vi "RegisterTrack.vi"(6 "Track ID":u64, 7 "Track Name":string, 8 "error in":errorcluster) -> (0 "error out":errorcluster)   [LabVIEW 2024, in "VS_Perfetto.lvlib"]
uses:
  VS_Perfetto.lvlib
  libvs_perfetto.dll
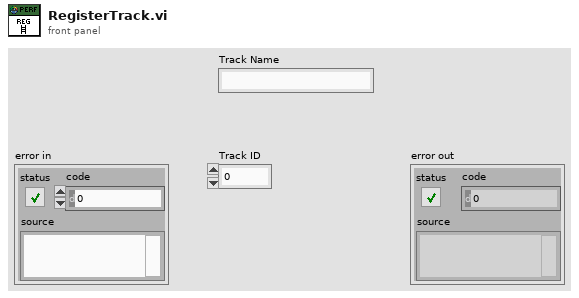
[diagram p1: front panel]
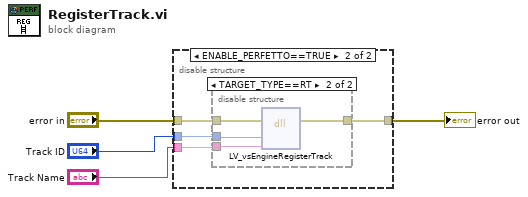
[diagram p0: block diagram]
diagram:
  n1 = disable-structure shown="ENABLE_PERFETTO==TRUE" {
    disable-tunnel: "Track Name" -> [_ w7]
    disable-tunnel: "error in" -> [w5 w8]
    disable-tunnel: [w5 w9] -> w3
    disable-tunnel: "Track ID" -> [_ w6]
    frame condition #0 (active) {
    }
    frame condition #1 {
      n2 = disable-structure shown="TARGET_TYPE==RT" {
        disable-tunnel: [w10 w14] -> w9
        disable-tunnel: w8 -> [w10 w13]
        disable-tunnel: w7 -> [_ w12]
        disable-tunnel: w6 -> [_ w11]
        frame condition #0 (active) {
        }
        frame condition #1 {
          n3 = dll-call lib="libvs_perfetto.*" fn="LV_vsEngineRegisterTrack"(error in=w13, "trackId"=w11, "trackName"=w12) -> (error out=w14:errorcluster)  [unwired: 5 in, 1 out]
        }
      }
    }
  }
  "error out" <- w3
